vi "电导率电极校准.vi"() -> ()   [LabVIEW 2016, in "斯坦道多参数.lvlib"]
uses:
  <vilib>/Utility/miscctls.llb/LVPointTypeDef.ctl
  <vilib>/Analysis/NI_AALBase.lvlib
panel:
  out "盐度":dbl caption="盐度测量值" format="%#.2g"
  out "温度":dbl format="%#.2g"
  out "当前信号值":dbl format="%#.2g"
  in  "校准停止":bool
  in  "校准启动":bool
  out "波形图表":sgl(graph) caption="历史曲线"
  out "第二点校准值":dbl
  out "第一点校准值":dbl
  in  "校准模式":enum16{"两点校准", "单点校准"}(ring)=enum."单点校准"
  out "提示":string
  out "最小值":sgl format="%#.2f"
  out "最大值":sgl format="%#.2f"
  out "mean":dbl caption="均值" format="%#.2f"
  out "standard deviation":dbl caption="标准差" format="%#.2f"
  out "变异系数":dbl format="%#.6f"
  out "标液2":dbl
  out "标液1":dbl
  out "当前读取值":dbl caption="当前测试值" format="%#.2g"
  out "电极系数":dbl
  out "偏移值补偿":dbl format="%#.2g"
  out "温度补偿系数":dbl caption="温度系数"
  # "电导率电极设定"
  # "请选择校准模式:"
  # "℃"
  # "uS/cm"
  # "uS/cm"
  # "cm"
  # "-1"
  # "uS/cm"
  # "%"
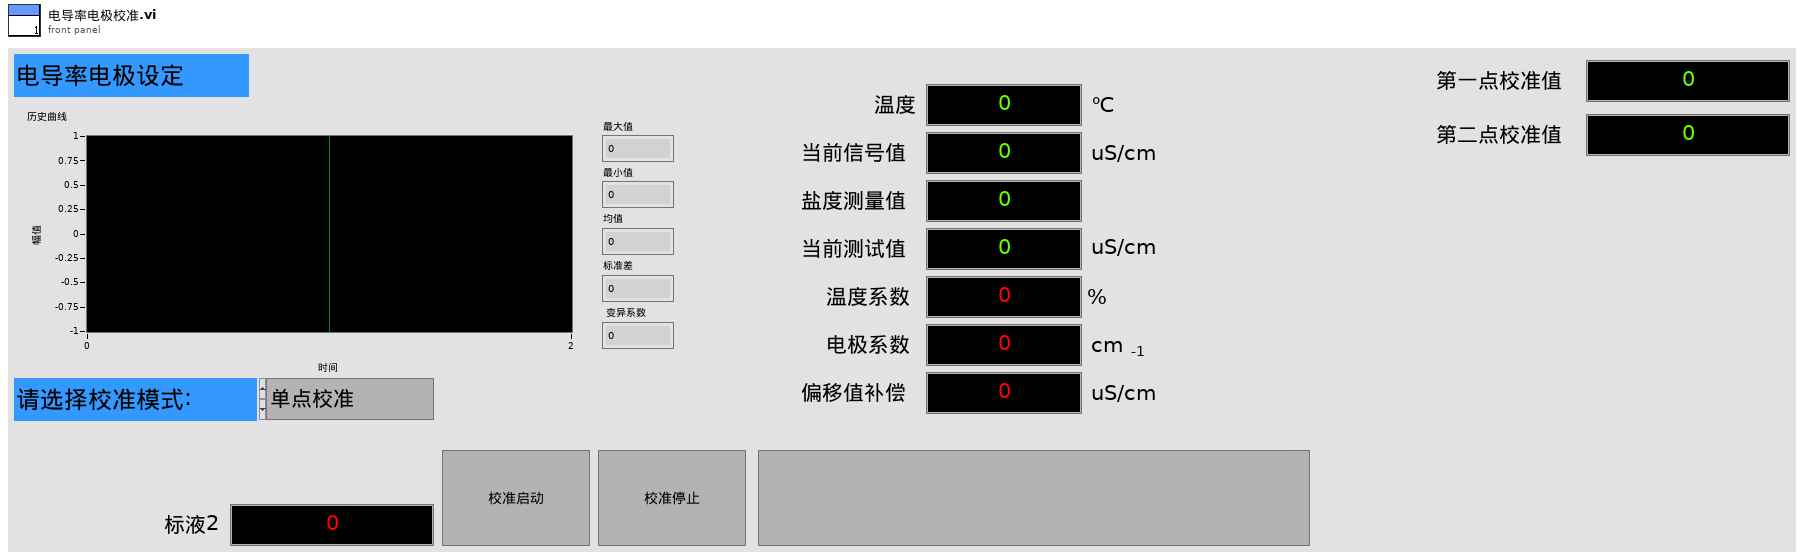
[diagram p1: front panel]
types:
  T1 = typedef "斯坦道多参数.lvlib/校准步骤.ctl" = enum16{"待机", "放置第一点标液", "第一点校准启动", "第一点校准写入", "第一点校准失败", "放置第二点标液", "第二点校准启动", "第二点校准写入", "第二点校准失败", "校准结果写入", "校准结束"}
  T2 = typedef "LVPointTypeDef.ctl" = cluster{"Horizontal":i16, "Vertical":i16}
  T3 = cluster{"电极状态标志":u16, "电极型号标志":u16, "电导率测量值":sgl, "温度测量值":sgl, "电导率信号值":sgl, "温度信号值":sgl, "温度补偿系数":sgl, "电导率偏移修正值":sgl, "温度偏移修正值":sgl, "手动温度补偿值":sgl, "电导率电极零点":sgl, "电导率电极斜率":sgl, "命令滤波设定":u16, "温度模式":enum16{"ATC", "MTC"}, "生产批次":u16, "电极序号":u16, "串口地址":u16, "串口波特率":enum16{"9600", "19200", "115200"}, "串口校验位":enum16{"NONE", "ODD", "EVEN"}, "串口停止位":enum16{"1bit", "2bit"}, "第一点标准值":sgl, "第二点标准值":sgl}
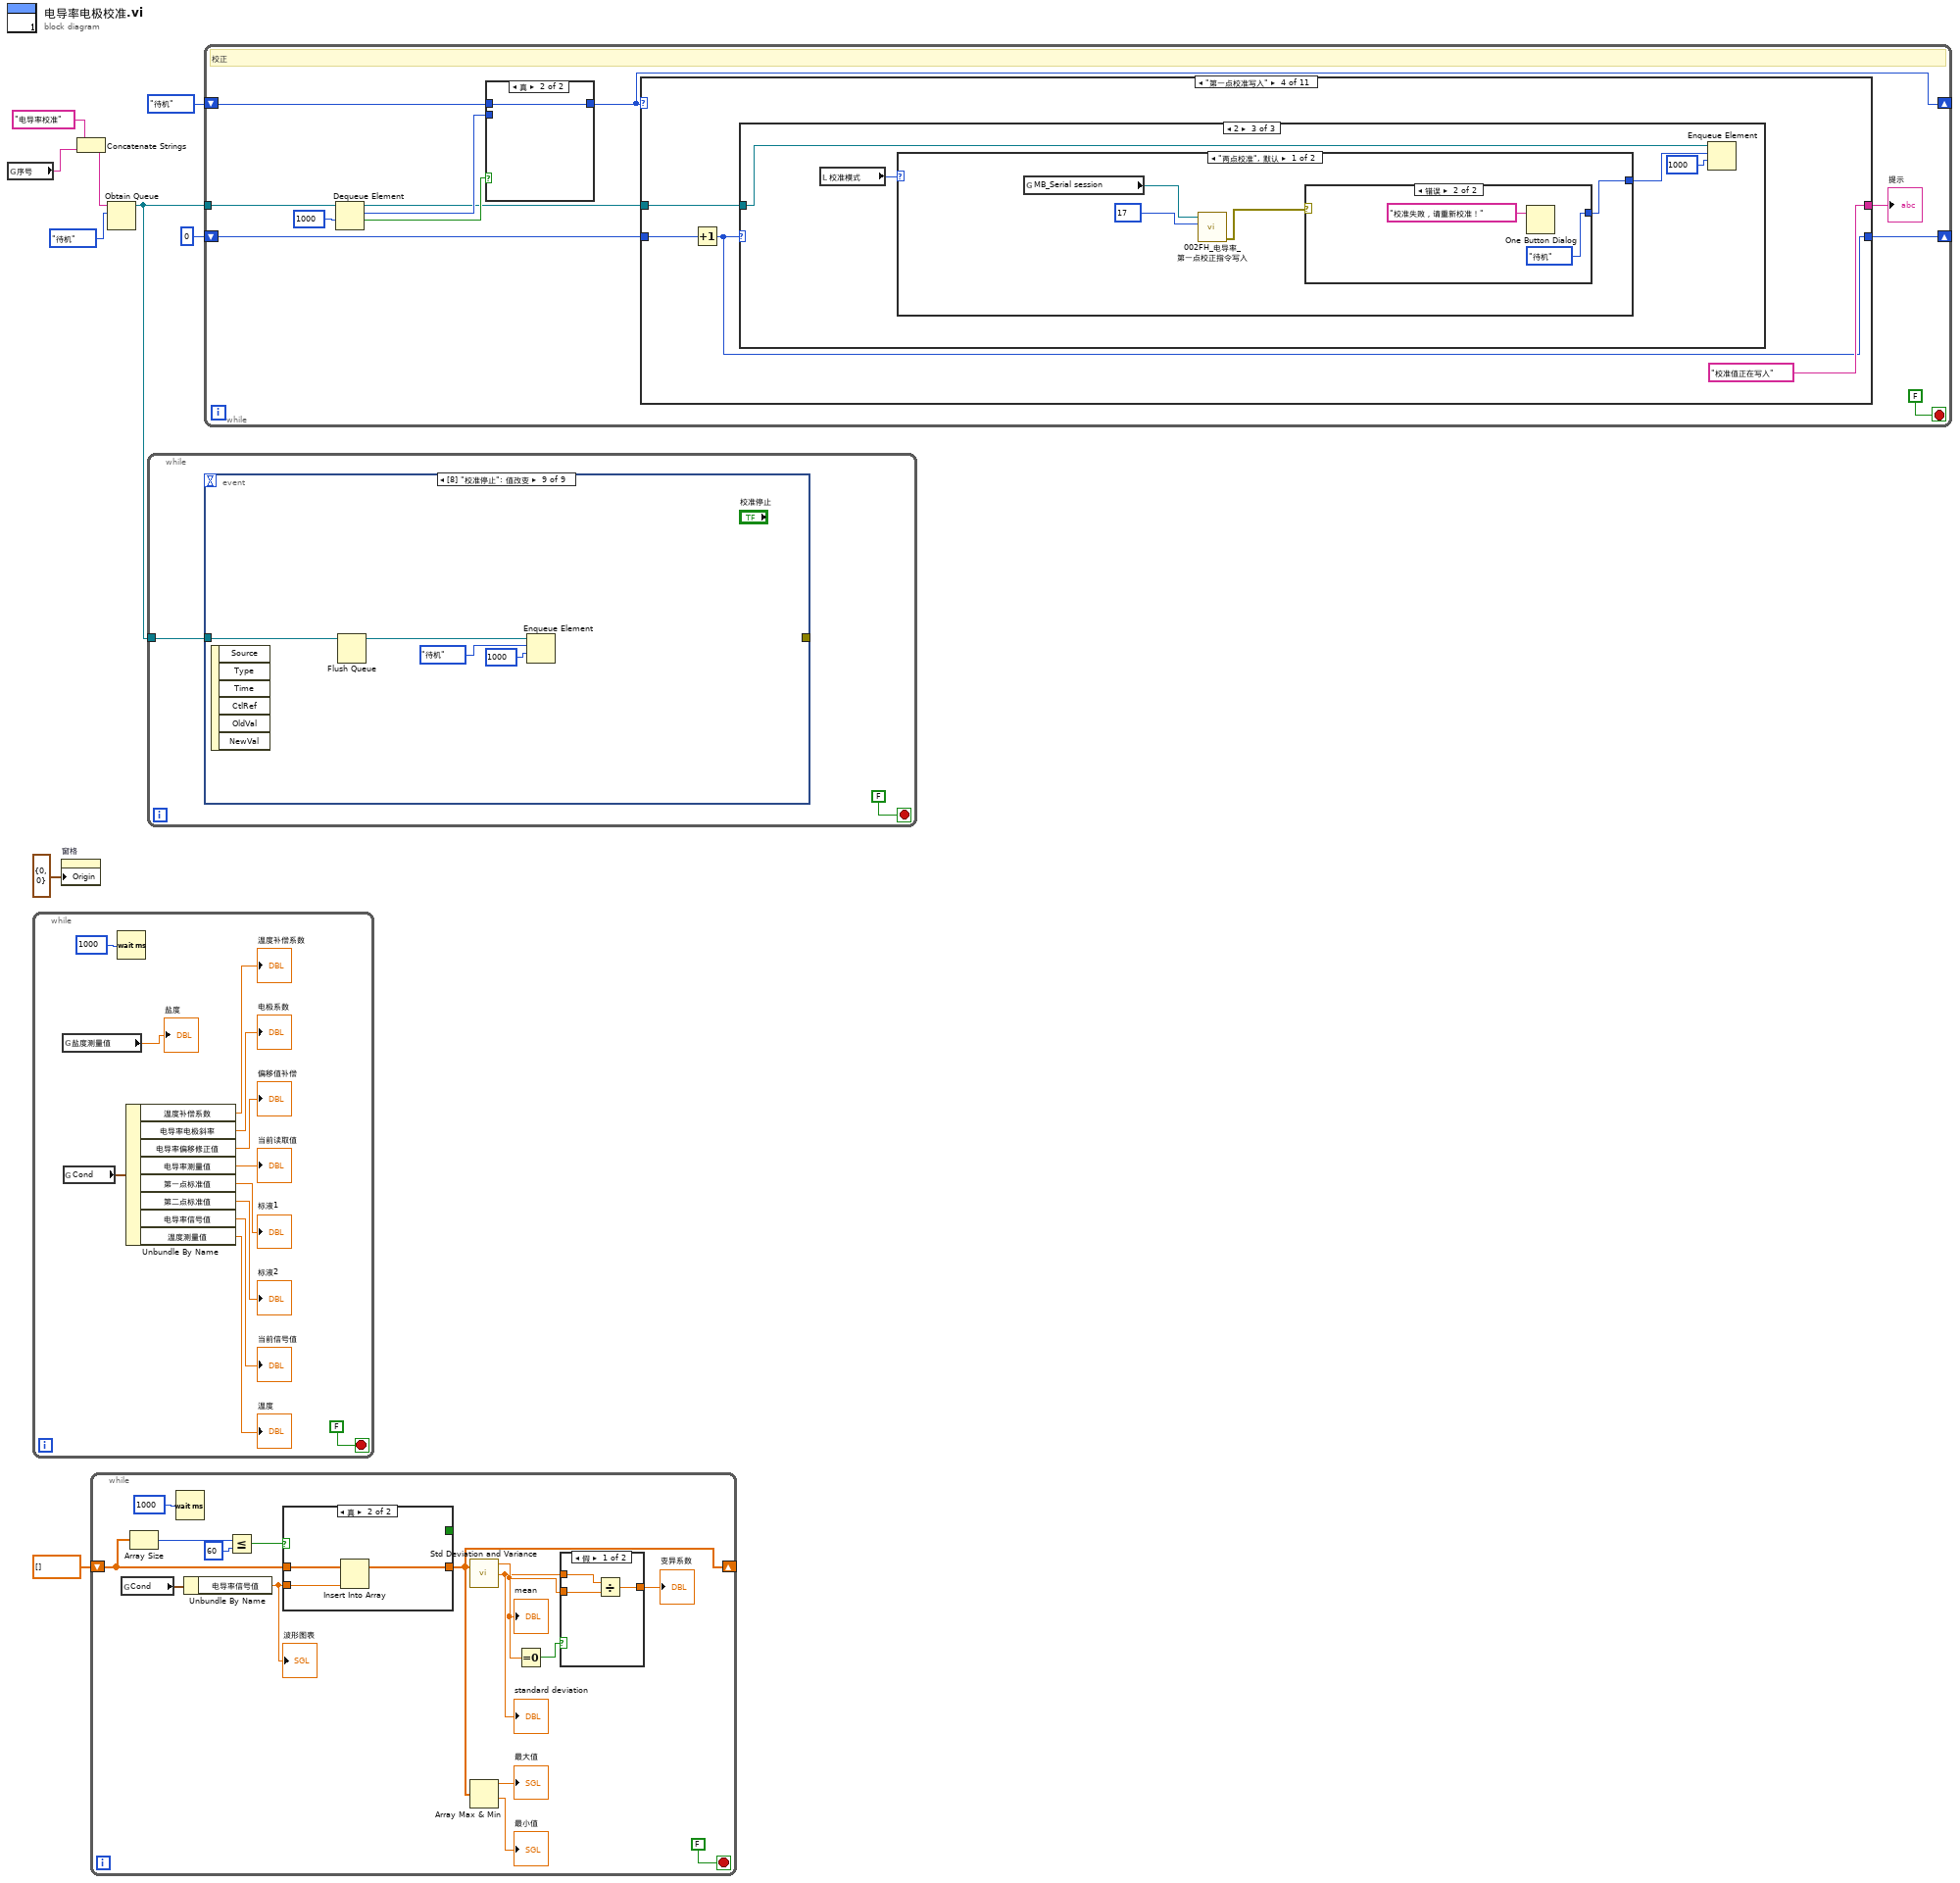
[diagram p0: block diagram]
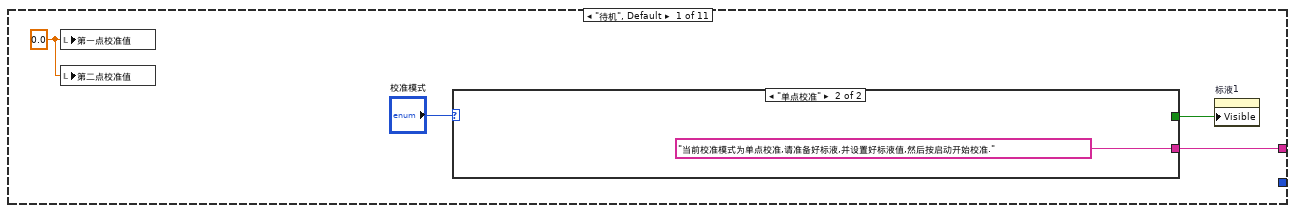
[diagram p3: hidden frame]
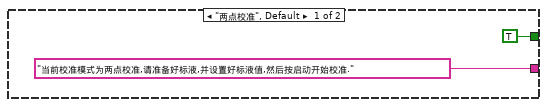
[diagram p4: hidden frame]
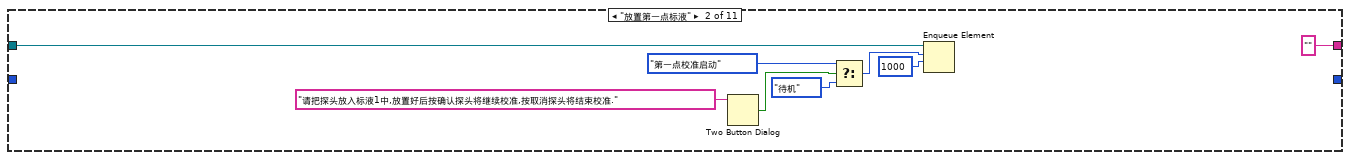
[diagram p5: hidden frame]
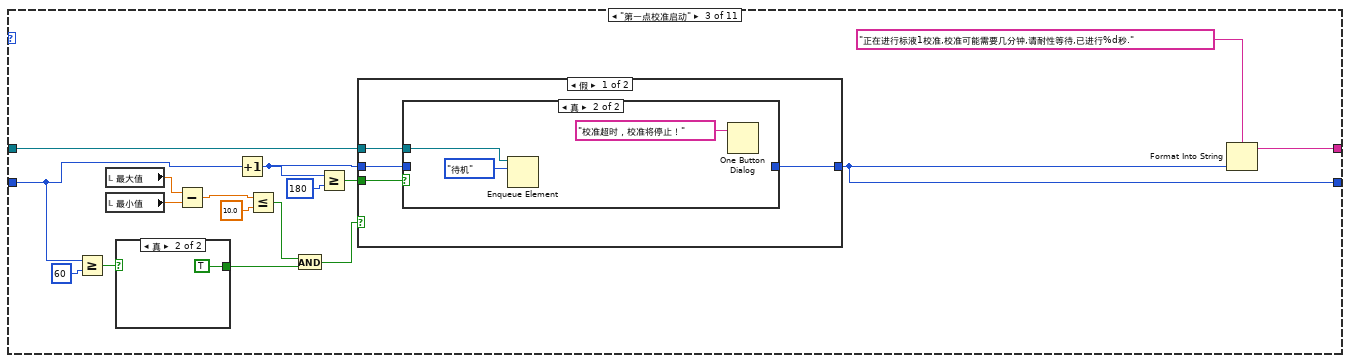
[diagram p6: hidden frame]
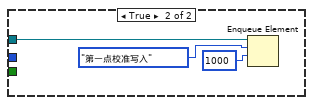
[diagram p8: hidden frame]
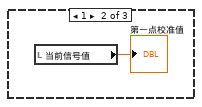
[diagram p11: hidden frame]
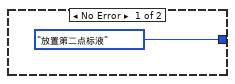
[diagram p12: hidden frame]
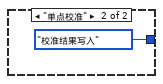
[diagram p13: hidden frame]
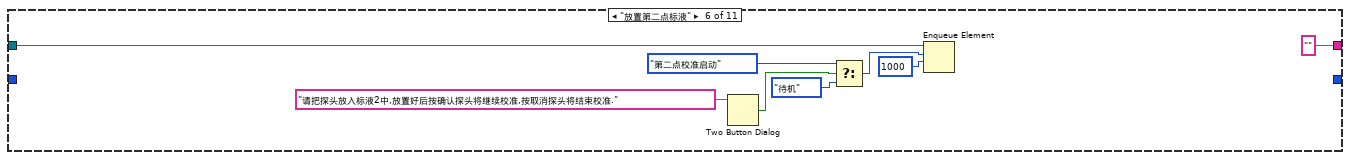
[diagram p15: hidden frame]
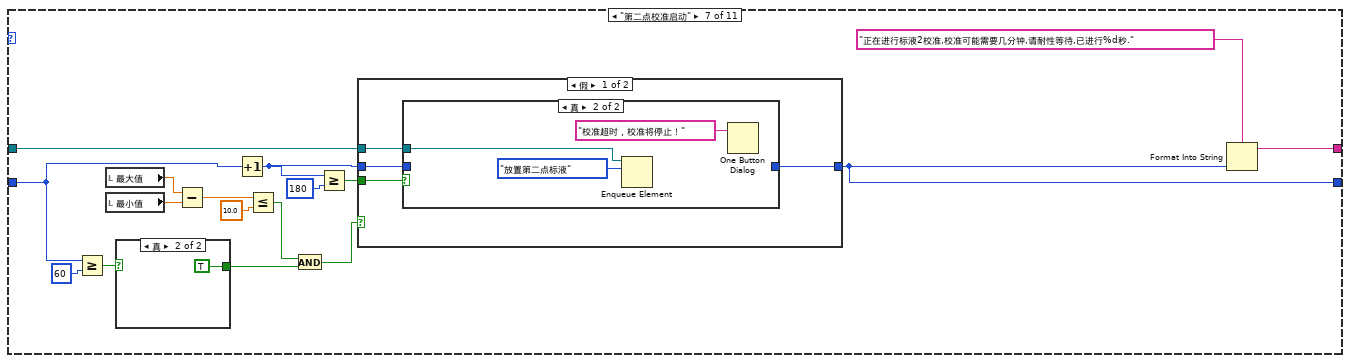
[diagram p16: hidden frame]
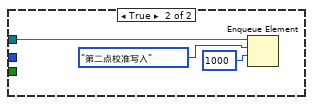
[diagram p18: hidden frame]
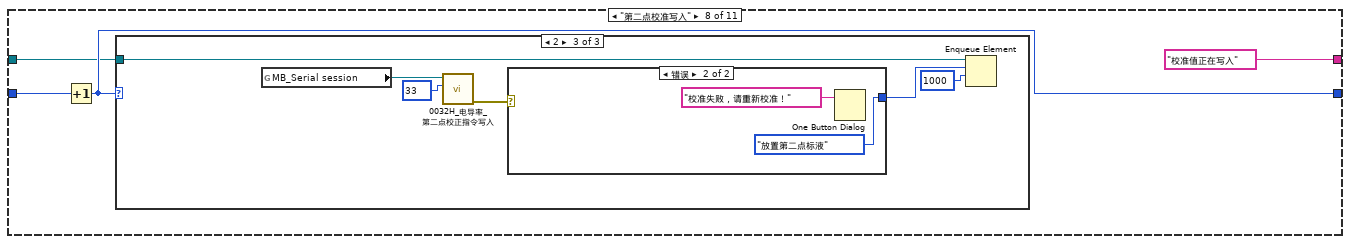
[diagram p20: hidden frame]
diagram:
  n1 = global read "多参数全局变量.vi" "序号"() -> (w1:string)
  n2 = while {
    stop <- FALSE stop-if-true
    n3 = global read "国弘过程全局变量.vi" "盐度测量值"() -> (→"盐度":sgl)
    n4 = global read "国弘过程全局变量.vi" "Cond"() -> (w19:T3)
    n5 = Wait (ms)(milliseconds to wait=u32 1000 ("等待时间（毫秒）")) -> ()  [unwired: 1 out]
    n6 = Unbundle By Name(w19) -> ("温度补偿系数"=→"温度补偿系数":sgl, "电导率电极斜率"=→"电极系数":sgl, "电导率偏移修正值"=→"偏移值补偿":sgl, "电导率测量值"=→"当前读取值":sgl, "第一点标准值"=→"标液1":sgl, "第二点标准值"=→"标液2":sgl, "电导率信号值"=→"当前信号值":sgl, "温度测量值"=→"温度":sgl)
  }
  n7 = property on="窗格" class="Pane"("Origin"=T2 {"Horizontal"=0, "Vertical"=0} ("原点")) -> ()  [unwired: 2 in, 2 out]
  n8 = Concatenate Strings("电导率校准" ("名称（未命名）"), w1) -> (w2:string)
  n9 = while {
    shift-right: [w25] -> _
    shift-left: sgl[] [] -> [w32]
    stop <- FALSE stop-if-true
    n10 = global read "国弘过程全局变量.vi" "Cond"() -> (w26:T3)
    n11 = Array Size(array=w32) -> (size(s)=w34:i32)
    n12 = Wait (ms)(milliseconds to wait=u32 1000 ("等待时间（毫秒）")) -> ()  [unwired: 1 out]
    n13 = Unbundle By Name(w26) -> ("电导率信号值"=w22:sgl)
    "波形图表" <- w22
    n14 = Less Or Equal?(x=w34, y=60) -> (x <= y?=w33:bool)
    n15 = case shown="真" w33 {
      tunnel: w32 -> [w45 w48]
      tunnel: w22 -> [w43 w47]
      tunnel: [w41 w46] -> w25
      tunnel: [TRUE _] -> _
      frame False {
        n16 = Replace Array Subset(array=w45, new element=w43) -> (w44:sgl[])  [unwired: 1 in]
        n17 = Rotate 1D Array(1:w44, 2:-1 ("n")) -> (0:w41:sgl[])
      }
      frame True {
        n18 = Insert Into Array(array=w48, new element=w47) -> (w46:sgl[])  [unwired: 1 in]
      }
    }
    n19 = call <vilib>:"Std Deviation and Variance.vi"("X"=w25) -> ("mean"=w30:dbl, "standard deviation"=w29:dbl)  [unwired: 1 in, 1 out]
    "mean" <- w30
    "standard deviation" <- w29
    n20 = Array Max & Min(array=w25) -> (max value=→"最大值":sgl, min value=→"最小值":sgl)  [unwired: 2 out]
    n21 = Equal To 0?(x=w30) -> (x = 0?=w31:bool)
    n22 = case shown="假" w31 {
      tunnel: w29 -> [w39 _]
      tunnel: [w38 _] -> w28
      tunnel: w30 -> [w37 _]
      frame False {
        n23 = Divide(x=w39, y=w37) -> (x/y=w38:dbl)
      }
      frame True {
      }
    }
    "变异系数" <- w28
  }
  n24 = Obtain Queue(name (unnamed)=w2, element data type=校准步骤."待机" ("枚举")) -> (queue out=w3:refnum<queue>)  [unwired: 3 in, 2 out]
  n25 = while {
    tunnel: w3 -> [w49]
    stop <- FALSE stop-if-true
    n26 = event shown="[8] \"校准停止\": 值改变" {
      selector: _ -> [_ _ _ _ _ _ _ _ _]
      dyn-events: _ -> [_ _ _ _ _ _ _ _ _]
      timeout: _ -> [_ _ _ _ _ _ _ _ _]
      tunnel: [_ _ w56 w59 w62 w66 w69 _ _] -> _
      tunnel: w49 -> [_ _ _ _ _ _ _ w72 w75]
      event Timeout {
        n27 = event-data() -> ()  [unwired: 1 in, 3 out]
      }
      event "偏移值补偿", "标液2", "电极系数", "温度补偿系数": Mouse Down {
        n28 = event-data() -> ("CtlRef"=w51:refnum<vi>)  [unwired: 1 in, 7 out]
        n29 = property class="DigNum (严格)"(reference=w51) -> (reference out=w52:refnum<vi>, "Value"=w53:dbl)  [unwired: 1 in, 1 out]
        n30 = call "数字键盘.vi"("OldNumber"=w53) -> ("NewNumber"=w54:sgl)
        n31 = property class="DigNum (严格)"(reference=w52, "Val(Sgnl)"=w54) -> ()  [unwired: 1 in, 2 out]
      }
      event "温度补偿系数": Value Change {
        n32 = event-data() -> ("NewVal"=w57:dbl)  [unwired: 1 in, 5 out]
        n33 = global read "多参数全局变量.vi" "MB_Serial session"() -> (w55:refnum<class "MB_Master_Serial.lvclass">)
        n34 = call "000AH_电导率_温度补偿系数写入.vi"("数值"=w57, "MB_Serial session in"=w55) -> ("error out"=w56:errorcluster)  [unwired: 8 in, 1 out]
      }
      event "偏移值补偿": Value Change {
        n35 = event-data() -> ("NewVal"=w60:dbl)  [unwired: 1 in, 5 out]
        n36 = global read "多参数全局变量.vi" "MB_Serial session"() -> (w58:refnum<class "MB_Master_Serial.lvclass">)
        n37 = call "000CH_电导率_电导率偏移修正值写入.vi"("数值"=w60, "MB_Serial session in"=w58) -> ("error out"=w59:errorcluster)  [unwired: 8 in, 1 out]
      }
      event "标液1": Value Change {
        n38 = event-data() -> ("NewVal"=w63:dbl)  [unwired: 1 in, 5 out]
        n39 = global read "多参数全局变量.vi" "MB_Serial session"() -> (w61:refnum<class "MB_Master_Serial.lvclass">)
        n40 = call "0030H_电导率_第一点标准值写入.vi"("数值"=w63, "MB_Serial session in"=w61) -> ("error out"=w62:errorcluster)  [unwired: 8 in, 1 out]
      }
      event "标液2": Value Change {
        n41 = event-data() -> ("NewVal"=w65:dbl)  [unwired: 1 in, 5 out]
        n42 = global read "多参数全局变量.vi" "MB_Serial session"() -> (w64:refnum<class "MB_Master_Serial.lvclass">)
        n43 = call "0033H_电导率_第二点标准值写入.vi"("数值"=w65, "MB_Serial session in"=w64) -> ("error out"=w66:errorcluster)  [unwired: 8 in, 1 out]
      }
      event "电极系数": Value Change {
        n44 = event-data() -> ("NewVal"=w68:dbl)  [unwired: 1 in, 5 out]
        n45 = global read "多参数全局变量.vi" "MB_Serial session"() -> (w67:refnum<class "MB_Master_Serial.lvclass">)
        n46 = call "0014H_电导率_电极系数写入.vi"("数值"=w68, "MB_Serial session in"=w67) -> ("error out"=w69:errorcluster)  [unwired: 8 in, 1 out]
      }
      event "校准启动": Value Change {
        n47 = event-data() -> ()  [unwired: 1 in, 6 out]
        n48 = local read "校准模式"() -> (w71:enum16{"两点校准", "单点校准"})
        n49 = case shown="\"两点校准\", 默认" w71 {
          tunnel: [校准步骤."放置第一点标液" ("元素") 校准步骤."放置第二点标液" ("元素")] -> w70
          frame "两点校准", Default {
          }
          frame "单点校准" {
          }
        }
        n50 = Enqueue Element(queue=w72, element=w70) -> ()  [unwired: 2 in, 3 out]
      }
      event "校准停止": Value Change {
        n51 = event-data() -> ()  [unwired: 1 in, 6 out]
        n52 = Flush Queue(queue=w75) -> (queue out=w76:refnum<queue>)  [unwired: 1 in, 2 out]
        n53 = Enqueue Element(queue=w76, element=校准步骤."待机" ("元素"), timeout in ms (-1)=1000 ("超时毫秒(-1)")) -> ()  [unwired: 1 in, 3 out]
      }
    }
  }
  n54 = while "While循环" {
    shift-right: [w80] -> _
    shift-left: 校准步骤."待机" ("枚举") -> [w81]
    shift-right: [w87] -> _
    shift-left: 0 -> [w88]
    tunnel: w3 -> [w85]
    stop <- FALSE stop-if-true
    # "校正"
    n55 = Dequeue Element(queue=w85, timeout in ms (-1)=1000 ("超时毫秒(-1)")) -> (queue out=w79:refnum<queue>, element=w82:T1, timed out?=w83:bool)  [unwired: 1 in, 1 out]
    n56 = case shown="真" w83 {
      tunnel: w82 -> [w90 _]
      tunnel: [w90 w91] -> w80
      tunnel: w81 -> [_ w91]
      frame False {
      }
      frame True {
      }
    }
    n57 = case shown="\"第一点校准写入\"" w80 {
      tunnel: [w95 "" ("提示") w122 "校准值正在写入" ("提示") _ "" ("提示") w176 "校准值正在写入" ("提示") _ w208 w219] -> w86
      tunnel: w88 -> [_ _ w116 w138 _ _ w170 w192 _ _ _]
      tunnel: [_ _ w107 w137 _ _ w161 w191 _ _ _] -> w87
      tunnel: w79 -> [_ w105 w110 w136 _ w159 w164 w190 _ w207 _]
      frame "待机", Default {
        w92 = 0.0 ("第一点校准值")
        n58 = local write "第一点校准值"(w92) -> ()
        n59 = local write "第二点校准值"(w92) -> ()
        n60 = case shown="\"单点校准\"" "校准模式" {
          tunnel: ["当前校准模式为两点校准,请准备好标液,并设置好标液值,然后按启动开始校准." ("提示") "当前校准模式为单点校准,请准备好标液,并设置好标液值,然后按启动开始校准." ("提示")] -> w95
          tunnel: [TRUE ("可见") _] -> w94
          frame "两点校准", Default {
          }
          frame "单点校准" {
          }
        }
        n61 = property on="标液1" class="DigNum (严格)"("Visible"=w94) -> ()  [unwired: 2 in, 2 out]
      }
      frame "放置第一点标液" {
        n62 = Two Button Dialog(message="请把探头放入标液1中,放置好后按确认探头将继续校准,按取消探头将结束校准." ("消息")) -> (T button?=w103:bool)  [unwired: 2 in]
        n63 = Select(t=校准步骤."第一点校准启动" ("元素"), s=w103, f=校准步骤."待机" ("元素")) -> (s? t:f=w100:T1)
        n64 = Enqueue Element(queue=w105, element=w100, timeout in ms (-1)=1000 ("超时毫秒(-1)")) -> ()  [unwired: 1 in, 3 out]
      }
      frame "第一点校准启动" {
        n65 = Greater Or Equal?(x=w116, y=60) -> (x >= y?=w117:bool)
        n66 = local read "最大值"() -> (w113:sgl)
        n67 = local read "最小值"() -> (w114:sgl)
        n68 = case shown="真" w117 {
          tunnel: [_ TRUE] -> w115
          frame False {
          }
          frame True {
          }
        }
        n69 = Subtract(x=w113, y=w114) -> (x-y=w112:sgl)
        n70 = Increment(x=w116) -> (x+1=w108:i32)
        n71 = Less Or Equal?(x=w112, y=10.0) -> (x <= y?=w120:bool)
        n72 = And(x=w120, y=w115) -> (x .and. y?=w111:bool)
        n73 = Greater Or Equal?(x=w108, y=180) -> (x >= y?=w109:bool)
        n74 = case shown="假" w111 {
          tunnel: w110 -> [w126 w134]
          tunnel: w109 -> [w127 _]
          tunnel: w108 -> [w125 _]
          tunnel: [w124 _] -> w107
          frame False {
            n75 = case shown="真" w127 {
              tunnel: w126 -> [_ w131]
              tunnel: w125 -> [w128 _]
              tunnel: [w128 _] -> w124
              frame False {
              }
              frame True {
                n76 = Enqueue Element(queue=w131, element=校准步骤."待机" ("元素")) -> ()  [unwired: 2 in, 3 out]
                n77 = One Button Dialog(message="校准超时，校准将停止！" ("消息")) -> ()  [unwired: 1 in, 1 out]
              }
            }
          }
          frame True {
            n78 = Enqueue Element(queue=w134, element=校准步骤."第一点校准写入" ("元素"), timeout in ms (-1)=1000 ("超时毫秒(-1)")) -> ()  [unwired: 1 in, 3 out]
          }
        }
        n79 = Format Into String(format string="正在进行标液1校准,校准可能需要几分钟,请耐性等待,已进行%d秒." ("格式字符串"), w107) -> (resulting string=w122:string)  [unwired: 2 in, 1 out]
      }
      frame "第一点校准写入" {
        n80 = Increment(x=w138) -> (x+1=w137:i32)
        n81 = case shown="2" w137 {
          tunnel: w136 -> [_ _ w144]
          frame 0, Default {
          }
          frame 1 {
            n82 = local read "当前信号值"() -> (→"第一点校准值":dbl)
          }
          frame 2 {
            n83 = local read "校准模式"() -> (w143:enum16{"两点校准", "单点校准"})
            n84 = case shown="\"两点校准\", 默认" w143 {
              tunnel: [w148 校准步骤."校准结果写入" ("元素")] -> w142
              frame "两点校准", Default {
                n85 = global read "多参数全局变量.vi" "MB_Serial session"() -> (w146:refnum<class "MB_Master_Serial.lvclass">)
                n86 = call "002FH_电导率_第一点校正指令写入.vi"("数值"=u16 17, "MB_Serial session in"=w146) -> ("error out"=w147:errorcluster)  [unwired: 8 in, 1 out]
                n87 = case shown="错误" w147 {
                  tunnel: [校准步骤."放置第二点标液" ("元素") 校准步骤."待机" ("元素")] -> w148
                  frame No Error {
                  }
                  frame Error {
                    n88 = One Button Dialog(message="校准失败，请重新校准！" ("消息")) -> ()  [unwired: 1 in, 1 out]
                  }
                }
              }
              frame "单点校准" {
              }
            }
            n89 = Enqueue Element(queue=w144, element=w142, timeout in ms (-1)=1000 ("超时毫秒(-1)")) -> ()  [unwired: 1 in, 3 out]
          }
        }
      }
      frame "第一点校准失败" {
      }
      frame "放置第二点标液" {
        n90 = Two Button Dialog(message="请把探头放入标液2中,放置好后按确认探头将继续校准,按取消探头将结束校准." ("消息")) -> (T button?=w157:bool)  [unwired: 2 in]
        n91 = Select(t=校准步骤."第二点校准启动" ("元素"), s=w157, f=校准步骤."待机" ("元素")) -> (s? t:f=w154:T1)
        n92 = Enqueue Element(queue=w159, element=w154, timeout in ms (-1)=1000 ("超时毫秒(-1)")) -> ()  [unwired: 1 in, 3 out]
      }
      frame "第二点校准启动" {
        n93 = Greater Or Equal?(x=w170, y=60) -> (x >= y?=w171:bool)
        n94 = local read "最大值"() -> (w167:sgl)
        n95 = local read "最小值"() -> (w168:sgl)
        n96 = case shown="真" w171 {
          tunnel: [_ TRUE] -> w169
          frame False {
          }
          frame True {
          }
        }
        n97 = Subtract(x=w167, y=w168) -> (x-y=w166:sgl)
        n98 = Increment(x=w170) -> (x+1=w162:i32)
        n99 = Less Or Equal?(x=w166, y=10.0) -> (x <= y?=w174:bool)
        n100 = And(x=w174, y=w169) -> (x .and. y?=w165:bool)
        n101 = Greater Or Equal?(x=w162, y=180) -> (x >= y?=w163:bool)
        n102 = case shown="假" w165 {
          tunnel: w164 -> [w180 w188]
          tunnel: w163 -> [w181 _]
          tunnel: w162 -> [w179 _]
          tunnel: [w178 _] -> w161
          frame False {
            n103 = case shown="真" w181 {
              tunnel: w180 -> [_ w185]
              tunnel: w179 -> [w182 _]
              tunnel: [w182 _] -> w178
              frame False {
              }
              frame True {
                n104 = Enqueue Element(queue=w185, element=校准步骤."放置第二点标液" ("元素")) -> ()  [unwired: 2 in, 3 out]
                n105 = One Button Dialog(message="校准超时，校准将停止！" ("消息")) -> ()  [unwired: 1 in, 1 out]
              }
            }
          }
          frame True {
            n106 = Enqueue Element(queue=w188, element=校准步骤."第二点校准写入" ("元素"), timeout in ms (-1)=1000 ("超时毫秒(-1)")) -> ()  [unwired: 1 in, 3 out]
          }
        }
        n107 = Format Into String(format string="正在进行标液2校准,校准可能需要几分钟,请耐性等待,已进行%d秒." ("格式字符串"), w161) -> (resulting string=w176:string)  [unwired: 2 in, 1 out]
      }
      frame "第二点校准写入" {
        n108 = Increment(x=w192) -> (x+1=w191:i32)
        n109 = case shown="2" w191 {
          tunnel: w190 -> [_ _ w200]
          frame 0, Default {
          }
          frame 1 {
            n110 = local read "当前信号值"() -> (→"第二点校准值":dbl)
          }
          frame 2 {
            n111 = global read "多参数全局变量.vi" "MB_Serial session"() -> (w197:refnum<class "MB_Master_Serial.lvclass">)
            n112 = call "0032H_电导率_第二点校正指令写入.vi"("数值"=u16 33, "MB_Serial session in"=w197) -> ("error out"=w195:errorcluster)  [unwired: 8 in, 1 out]
            n113 = case shown="错误" w195 {
              tunnel: [校准步骤."校准结果写入" ("元素") 校准步骤."放置第二点标液" ("元素")] -> w198
              frame No Error {
              }
              frame Error {
                n114 = One Button Dialog(message="校准失败，请重新校准！" ("消息")) -> ()  [unwired: 1 in, 1 out]
              }
            }
            n115 = Enqueue Element(queue=w200, element=w198, timeout in ms (-1)=1000 ("超时毫秒(-1)")) -> ()  [unwired: 1 in, 3 out]
          }
        }
      }
      frame "第二点校准失败" {
      }
      frame "校准结果写入" {
        n116 = Enqueue Element(queue=w207, element=校准步骤."校准结束" ("元素")) -> ()  [unwired: 2 in, 3 out]
        n117 = global read "国弘过程全局变量.vi" "Cond"() -> (w205:T3)
        n118 = Unbundle By Name(w205) -> ("电极状态标志"=w204:u16)
        n119 = case shown="0, 默认" w204 {
          tunnel: [w210 "校准失败"] -> w208
          frame 0, Default {
            n120 = local read "校准模式"() -> (w209:enum16{"两点校准", "单点校准"})
            n121 = case shown="\"单点校准\"" w209 {
              tunnel: [w211 w215] -> w210
              frame "两点校准", Default {
                n122 = local read "第一点校准值"() -> (w213:dbl)
                n123 = local read "第二点校准值"() -> (w214:dbl)
                n124 = Format Into String(format string="两点校准结果：\n第一点校准值：%f\n第二点校准值：%f" ("提示"), w213, w214) -> (resulting string=w211:string)  [unwired: 2 in, 1 out]
              }
              frame "单点校准" {
                n125 = local read "第二点校准值"() -> (w217:dbl)
                n126 = Format Into String(format string="校准结果：\n校准值：%f" ("提示"), w217) -> (resulting string=w215:string)  [unwired: 2 in, 1 out]
              }
            }
          }
          frame 3, 4 {
          }
        }
        n127 = One Button Dialog(message=w208) -> ()  [unwired: 1 in, 1 out]
      }
      frame "校准结束" {
        n128 = local read "提示"() -> (w219:string)
      }
    }
    "提示" <- w86
  }
